vi "Get Used Encoding.vi"(8 "error in (no error)":errorcluster, 11 "CConfig Automatic Encoding in":refnum<class "CConfig Automatic Encoding.lvclass">) -> (0 "error out":errorcluster, 3 "CConfig Encoding out":refnum<class "CConfig Encoding.lvclass">)   [LabVIEW 2013, in "CConfig Automatic Encoding.lvclass"]
doc: "Copyright 2018, Carya Automatisering, Wiebe Walstra."
uses:
  CConfig Automatic Encoding.lvclass
  CConfig Encoding.lvclass
  CConfig Automatic Encoding.lvclass/CConfig Automatic Encoding.ctl
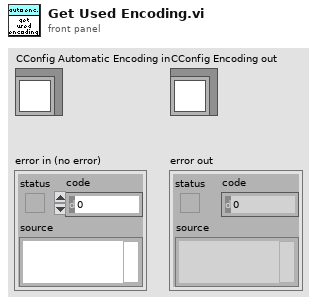
[diagram p1: front panel]
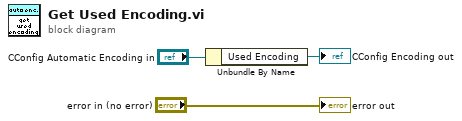
[diagram p0: block diagram]
diagram:
  n1 = Unbundle By Name("CConfig Automatic Encoding in") -> ("Used Encoding"=→"CConfig Encoding out":refnum<class "CConfig Encoding.lvclass">)
  "error out" <- "error in (no error)"
